vi "Init.vi"(8 "error in (no error)":errorcluster) -> (0 "error out":errorcluster)   [LabVIEW 2015, in "App Config.lvlib"]
uses:
  App Config.lvlib
  FGV Action.ctl
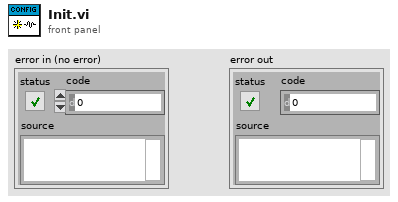
[diagram p1: front panel]
types:
  T1 = typedef "App Config.lvlib/FGV Action.ctl" = enum16{"Read", "Write"}
  T2 = typedef "App Config.lvlib/App Config Data.ctl" = cluster{"Music Folder Path":path, "Temp Images Path":path}
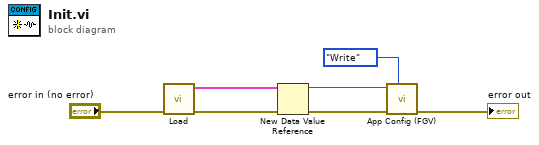
[diagram p0: block diagram]
diagram:
  n1 = call "Load.vi"("error in (no error)"="error in (no error)") -> ("error out"=w5:errorcluster, "App Config Data Out"=w4:T2)  [unwired: 9 in]
  n2 = New Data Value Reference(data value=w4, error in=w5) -> (data value reference=w3:refnum<data-value>, error out=w6:errorcluster)
  n3 = call "App Config (FGV).vi"("Action (Read)"=FGV_Action."Write", "error in (no error)"=w6, "DVR In"=w3) -> ("error out"=→"error out":errorcluster)  [unwired: 7 in, 1 out]
